vi "DHE_DEfaultInterlock.vi"(9 "field":string, 10 "parent":string, 11 "DHE_ImgState":T1(ring)) -> (2 "interlock":bool)   [LabVIEW 2016]
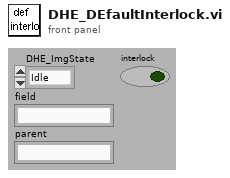
[diagram p1: front panel]
types:
  T1 = enum16{"Idle", "Exposing", "Paused", "AbortExp", "Reading", "AbortRead", "FinishedReading", "Resetting", "Reducing", "Initializing"}
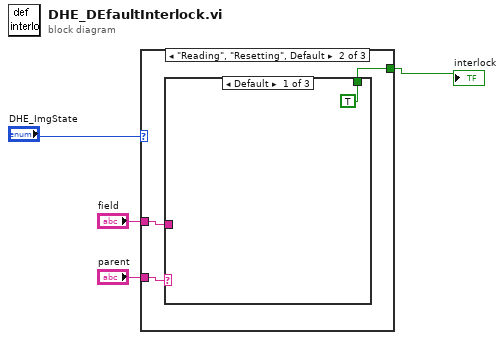
[diagram p0: block diagram]
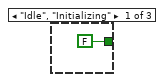
[diagram p2: hidden frame]
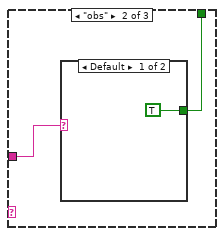
[diagram p3: hidden frame]
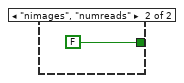
[diagram p4: hidden frame]
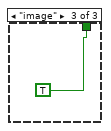
[diagram p5: hidden frame]
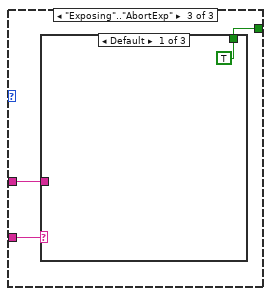
[diagram p6: hidden frame]
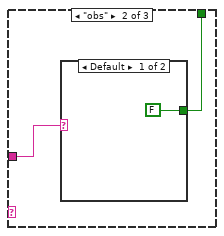
[diagram p7: hidden frame]
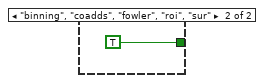
[diagram p8: hidden frame]
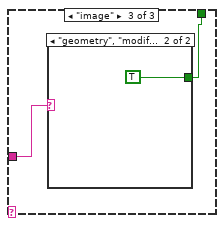
[diagram p9: hidden frame]
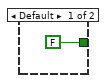
[diagram p10: hidden frame]
diagram:
  n1 = case shown="\"Reading\", \"Resetting\", Default" "DHE_ImgState" {
    tunnel: [FALSE ("status") w6 w16] -> w1
    tunnel: "parent" -> [_ w8 w17]
    tunnel: "field" -> [_ w7 w15]
    frame "Idle", "Initializing" {
    }
    frame "Reading", "Resetting", Default {
      n2 = case shown="Default" w8 {
        tunnel: [TRUE w11 TRUE] -> w6
        tunnel: w7 -> [_ w10 _]
        frame Default {
        }
        frame "obs" {
          n3 = case shown="Default" w10 {
            tunnel: [TRUE FALSE] -> w11
            frame Default {
            }
            frame "nimages", "numreads" {
            }
          }
        }
        frame "image" {
        }
      }
    }
    frame "Exposing".."AbortExp" {
      n4 = case shown="Default" w17 {
        tunnel: [TRUE w20 w23] -> w16
        tunnel: w15 -> [_ w19 w24]
        frame Default {
        }
        frame "obs" {
          n5 = case shown="Default" w19 {
            tunnel: [FALSE TRUE] -> w20
            frame Default {
            }
            frame "binning", "coadds", "fowler", "roi", "sur" {
            }
          }
        }
        frame "image" {
          n6 = case shown="\"geometry\", \"modifiers\"" w24 {
            tunnel: [FALSE TRUE] -> w23
            frame Default {
            }
            frame "geometry", "modifiers" {
            }
          }
        }
      }
    }
  }
  "interlock" <- w1
